vi "Flag Array to Error Message.vi"(6 "Verbose Message Array":string[](array[string]), 8 "Error In":errorcluster, 9 "OK Message":string, 10 "Message Array":string[](array[string]), 11 "Flag Array":bool[](array[boolean])) -> (0 "Error Out":errorcluster, 1 "Verbose Message":string, 2 "Message":string, 3 "Flag OR":bool)   [LabVIEW 2019]
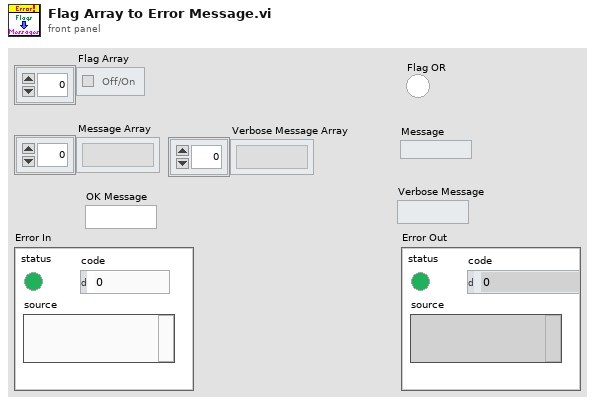
[diagram p1: front panel]
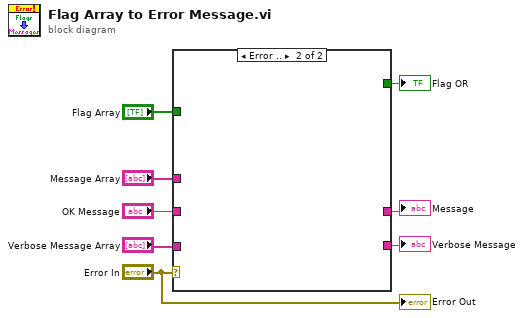
[diagram p0: block diagram]
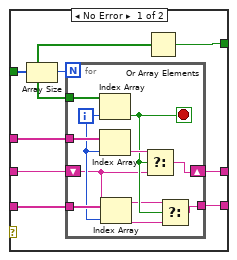
[diagram p2: hidden frame]
diagram:
  n1 = case shown="Error .." "Error In" {
    tunnel: [w16 _] -> w8
    tunnel: "OK Message" -> [w14 _]
    tunnel: [w13 _] -> w6
    tunnel: "Flag Array" -> [w10 _]
    tunnel: "Message Array" -> [w12 _]
    tunnel: "Verbose Message Array" -> [w11 _]
    tunnel: [w9 _] -> w1
    frame No Error {
      n2 = Array Size(array=w10) -> (size(s)=w15:i32)
      n3 = for {
        N: w15 -> [_]
        shift-right: [w23] -> w13
        shift-left: w14 -> [w18]
        tunnel: w10 -> [w26]
        tunnel: w12 -> [w25]
        tunnel: w11 -> [w22]
        tunnel: [w17] -> w9
        i -> [w21]
        stop <- w20 stop-if-true
        n4 = Index Array(array=w26, index=w21) -> (element=w20:bool)
        n5 = Index Array(array=w25, index=w21) -> (element=w24:string)
        n6 = Index Array(array=w22, index=w21) -> (element=w19:string)
        n7 = Select(t=w24, s=w20, f=w18) -> (s? t:f=w23:string)
        n8 = Select(t=w19, s=w20, f=w18) -> (s? t:f=w17:string)
      }
      n9 = Or Array Elements(Boolean array=w10) -> (logical OR=w16:bool)
    }
    frame Error {
    }
  }
  "Verbose Message" <- w1
  "Message" <- w6
  "Flag OR" <- w8
  "Error Out" <- "Error In"
